vi "Validate Incoming Packet.vi"(8 "error in (no error)":errorcluster, 10 "ControlPacket":refnum<class "ControlPacket.lvclass">, 11 "Session.Server in":refnum<class "Session.Server.lvclass">) -> (0 "error out":errorcluster, 2 "ControlPacket out":refnum<class "ControlPacket.lvclass">, 3 "Session.Server out":refnum<class "Session.Server.lvclass">)   [LabVIEW 2013, in "MQTT Server.lvlib" / "Session.Server.lvclass"]
uses:
  Session.Server.lvclass
  <vilib>/LabVIEW Open Source Project/MQTT Control Packets/Control Packets/ControlPacket/ControlPacket.lvclass
  Session.Server.lvclass/Session.Server.ctl
  <vilib>/LabVIEW Open Source Project/MQTT Control Packets/Control Packets/CONNECT/CONNECT.lvclass
  <vilib>/LabVIEW Open Source Project/MQTT Connection/MQTT_Base/Session/Session.lvclass/Session.ctl
  <vilib>/LabVIEW Open Source Project/MQTT Connection/MQTT_Base/Session/Session.lvclass
  <vilib>/LabVIEW Open Source Project/MQTT Control Packets/Control Packets/SUBSCRIBE/SUBSCRIBE.lvclass
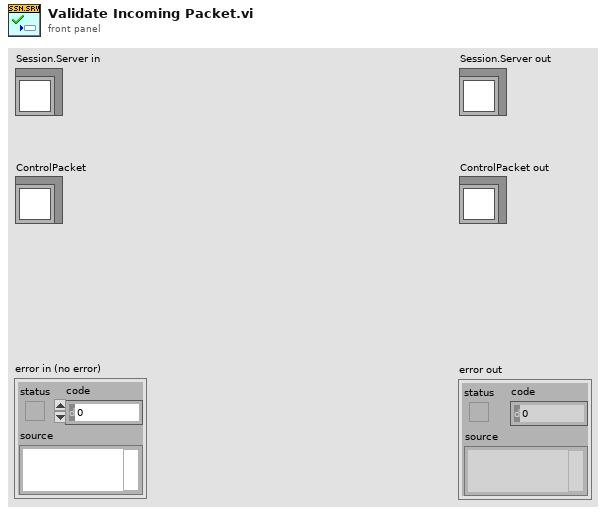
[diagram p1: front panel]
types:
  T1 = typedef "MQTT_Control_Packets.lvlib/ControlPacket.lvclass/Control Packet Type -- enum.ctl" = enum16{"Reserved", "CONNECT", "CONNACK", "PUBLISH", "PUBACK", "PUBREC", "PUBREL", "PUBCOMP", "SUBSCRIBE", "SUBACK", "UNSUBSCRIBE", "UNSUBACK", "PINGREQ", "PINGRESP", "DISCONNECT", "AUTH"}
  T2 = typedef "MQTT_Control_Packets.lvlib/SUBSCRIBE.lvclass/Topic Subscription -- cluster.ctl" = cluster{"Topic Filter":string, "QoS":T3}
  T3 = typedef "MQTT_Control_Packets.lvlib/ControlPacket.lvclass/QualityOfService -- enum.ctl" = enum16{"0 (At Most Once)", "1 (At Least Once)", "2 (Exactly Once)"}
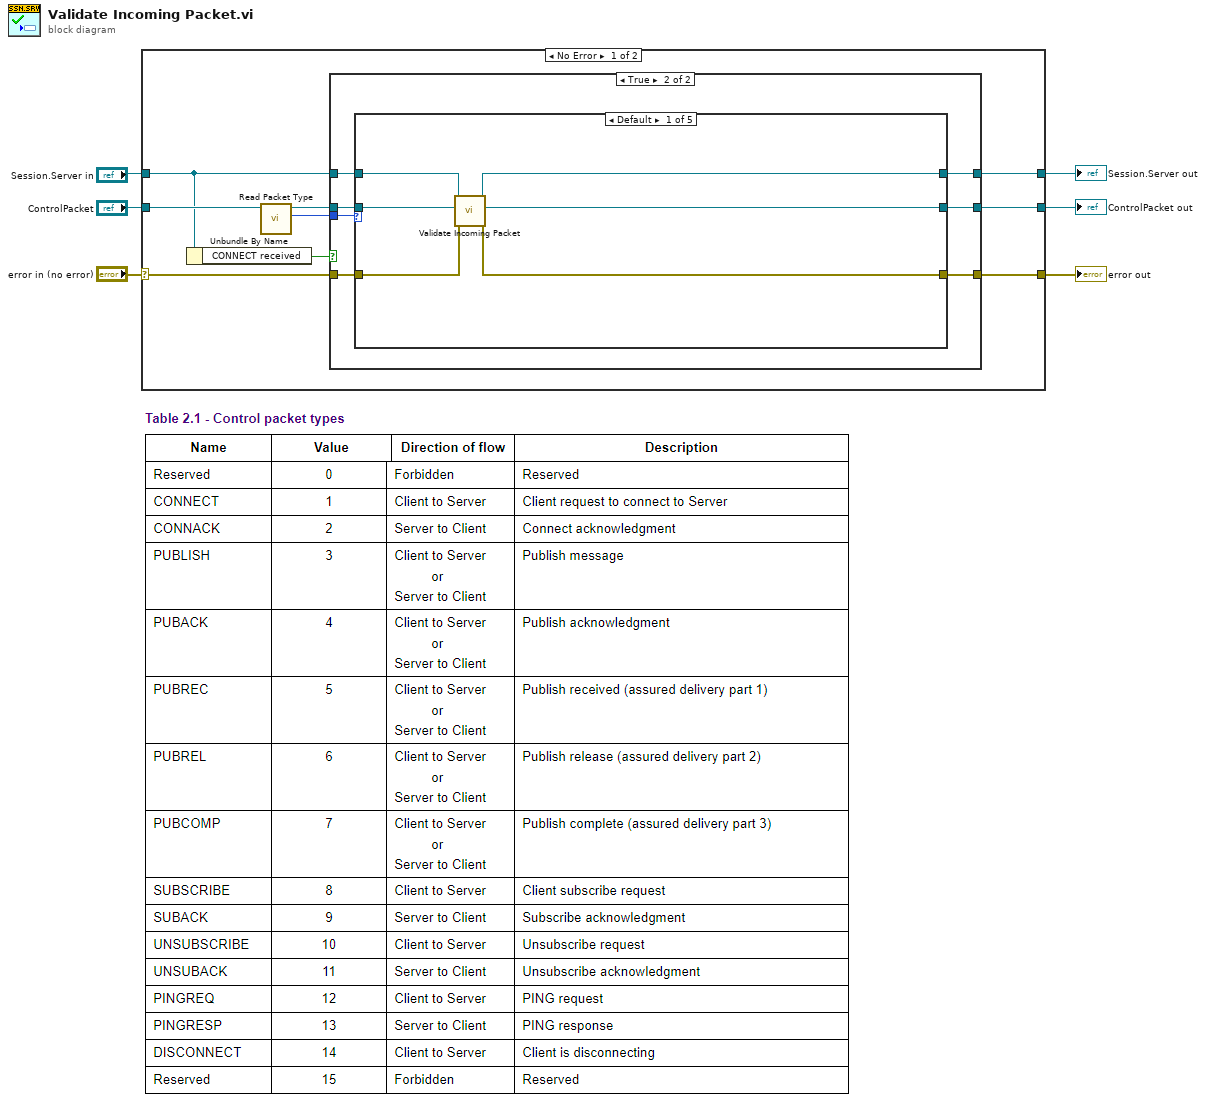
[diagram p0: block diagram]
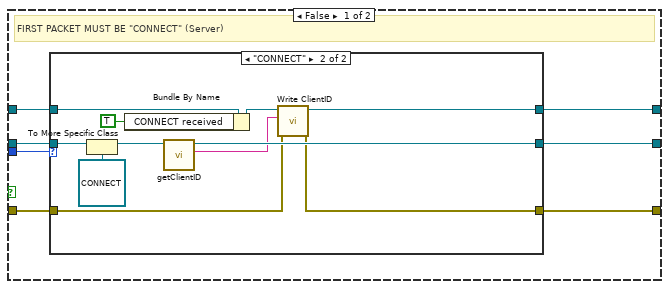
[diagram p2: hidden frame]
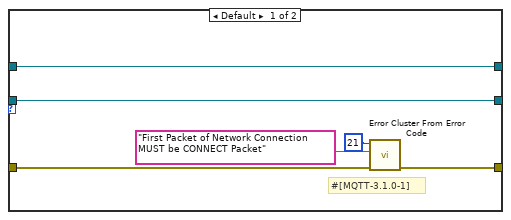
[diagram p3: hidden frame]
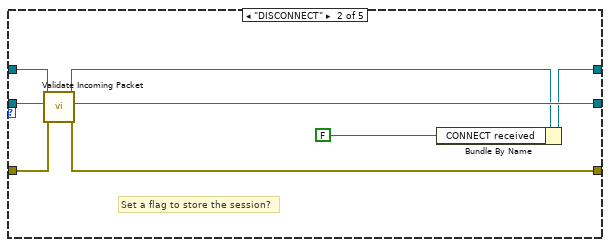
[diagram p4: hidden frame]
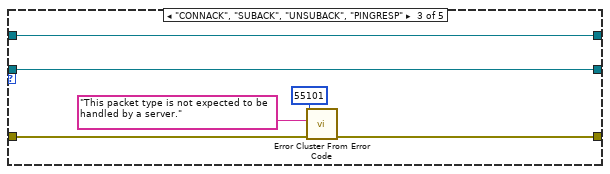
[diagram p5: hidden frame]
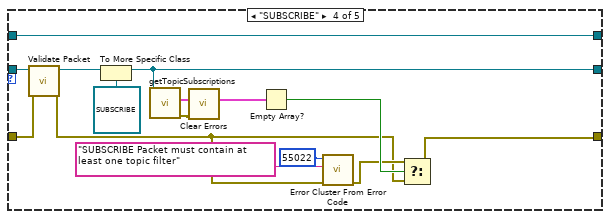
[diagram p6: hidden frame]
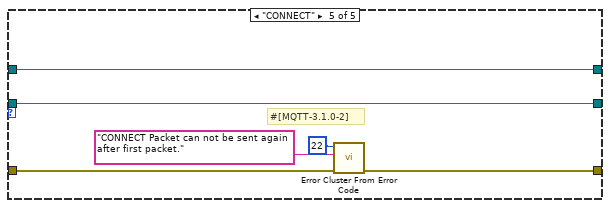
[diagram p7: hidden frame]
diagram:
  n1 = case shown="No Error" "error in (no error)" {
    selector: "error in (no error)" -> [w12 w89]
    tunnel: [w11 w89] -> w1
    tunnel: [w13 w88] -> w3
    tunnel: "Session.Server in" -> [w10 w88]
    tunnel: "ControlPacket" -> [w14 w87]
    tunnel: [w15 w87] -> w2
    frame No Error {
      n2 = Unbundle By Name(w10) -> ("CONNECT received"=w9:bool)
      n3 = call <vilib>:"Read Packet Type.vi"("ControlPacket in"=w14) -> ("Control Packet Type"=w7:T1, "ControlPacket out"=w8:refnum<class "ControlPacket.lvclass">)  [unwired: 9 in]
      n4 = case shown="True" w9 {
        tunnel: w8 -> [w16 w45]
        tunnel: [w17 w44] -> w15
        tunnel: w10 -> [w19 w41]
        tunnel: w7 -> [w20 w46]
        tunnel: [w18 w40] -> w13
        tunnel: w12 -> [w22 w43]
        tunnel: [w21 w42] -> w11
        frame False {
          # "FIRST PACKET MUST BE \"CONNECT\" (Server)"
          n5 = case shown="\"CONNECT\"" w20 {
            tunnel: w22 -> [w27 w31]
            tunnel: [w28 w32] -> w21
            tunnel: w19 -> [w26 w39]
            tunnel: [w26 w35] -> w18
            tunnel: [w25 w33] -> w17
            tunnel: w16 -> [w25 w36]
            frame Default {
              # "#[MQTT-3.1.0-1]"
              n6 = call <vilib>:"Error Cluster From Error Code.vi"("error in (no error)"=w27, "error message (\"\")"="First Packet of Network Connection MUST be CONNECT Packet", "error code (0)"=21) -> ("error out"=w28:errorcluster)  [unwired: 6 in]
            }
            frame "CONNECT" {
              n7 = To More Specific Class(target class=refnum<class "CONNECT.lvclass"> refnum ("CONNECT.lvclass"), reference=w36) -> (specific class reference=w29:refnum<class "CONNECT.lvclass">)  [unwired: 1 in, 1 out]
              n8 = Bundle By Name(cluster=w39, "CONNECT received"=TRUE) -> (w34:refnum<class "Session.Server.lvclass">)
              n9 = call <vilib>:"getClientID.vi"("CONNECT in"=w29) -> ("Client ID"=w30:string, "CONNECT out"=w33:refnum<class "CONNECT.lvclass">)  [unwired: 9 in]
              n10 = call <vilib>:"Write ClientID.vi"("error in (no error)"=w31, "Client ID"=w30, "Session in"=w34) -> ("error out"=w32:errorcluster, "Session out"=w35:refnum<class "Session.Server.lvclass">)  [unwired: 7 in]
            }
          }
        }
        frame True {
          n11 = case shown="Default" w46 {
            tunnel: w45 -> [w52 w60 w65 w70 w84]
            tunnel: [w51 w59 w65 w79 w84] -> w44
            tunnel: w43 -> [w49 w57 w62 w68 w83]
            tunnel: [w48 w56 w63 w71 w82] -> w42
            tunnel: w41 -> [w50 w58 w66 w72 w81]
            tunnel: [w47 w53 w66 w72 w81] -> w40
            frame Default {
              n12 = call-parent "Validate Incoming Packet.vi"("error in (no error)"=w49, "ControlPacket"=w52, "Session in"=w50) -> ("error out"=w48:errorcluster, "ControlPacket out"=w51:refnum<class "ControlPacket.lvclass">, "Session out"=w47:refnum<class "Session.Server.lvclass">)  [unwired: 6 in]
            }
            frame "DISCONNECT" {
              # "Set a flag to store the session?"
              n13 = call-parent "Validate Incoming Packet.vi"("error in (no error)"=w57, "ControlPacket"=w60, "Session in"=w58) -> ("error out"=w56:errorcluster, "ControlPacket out"=w59:refnum<class "ControlPacket.lvclass">, "Session out"=w54:refnum<class "Session.Server.lvclass">)  [unwired: 6 in]
              n14 = Bundle By Name(cluster=w54, "CONNECT received"=FALSE) -> (w53:refnum<class "Session.Server.lvclass">)
            }
            frame "CONNACK", "SUBACK", "UNSUBACK", "PINGRESP" {
              n15 = call <vilib>:"Error Cluster From Error Code.vi"("error in (no error)"=w62, "error message (\"\")"="This packet type is not expected to be handled by a server.", "error code (0)"=55101) -> ("error out"=w63:errorcluster)  [unwired: 6 in]
            }
            frame "SUBSCRIBE" {
              n16 = call <vilib>:"Validate Packet.vi"("error in (no error)"=w68, "ControlPacket in"=w70) -> ("error out"=w67:errorcluster, "ControlPacket out"=w69:refnum<class "ControlPacket.lvclass">)  [unwired: 8 in]
              n17 = To More Specific Class(target class=refnum<class "SUBSCRIBE.lvclass"> refnum ("SUBSCRIBE.lvclass"), reference=w69) -> (specific class reference=w79:refnum<class "SUBSCRIBE.lvclass">)  [unwired: 1 in, 1 out]
              n18 = call <vilib>:"getTopicSubscriptions.vi"("SUBSCRIBE in"=w79) -> ("error out"=w73:errorcluster, "Topic Subscriptions"=w78:T2[])  [unwired: 8 in, 1 out]
              n19 = call <vilib>:"Clear Errors.vi"("error in (no error)"=w73) -> ()  [unwired: 6 in, 1 out]
              n20 = Empty Array?(array=w78) -> (empty?=w75:bool)
              n21 = call <vilib>:"Error Cluster From Error Code.vi"("error in (no error)"=w67, "error message (\"\")"="SUBSCRIBE Packet must contain at least one topic filter", "error code (0)"=55022) -> ("error out"=w74:errorcluster)  [unwired: 6 in]
              n22 = Select(t=w74, s=w75, f=w67) -> (s? t:f=w71:errorcluster)
            }
            frame "CONNECT" {
              # "#[MQTT-3.1.0-2]"
              n23 = call <vilib>:"Error Cluster From Error Code.vi"("error in (no error)"=w83, "error message (\"\")"="CONNECT Packet can not be sent again after first packet.", "error code (0)"=22) -> ("error out"=w82:errorcluster)  [unwired: 6 in]
            }
          }
        }
      }
    }
    frame Error {
    }
  }
  "error out" <- w1
  "Session.Server out" <- w3
  "ControlPacket out" <- w2
